vi "Stage Finished Playback.vi"(8 "error in (no error)":errorcluster, 11 "Internal Vars":T1={"Test_File"="", "Status"="Done", "RF_Center_Freq"="0", "RF_Gain"="0", "BB_Gain"="0", "Error"="", "file_max"="0", "file_index"="0"}) -> (0 "error out":errorcluster)   [LabVIEW 2017]
uses:
  TypeDef/RF Internal Data Structure (string).ctl
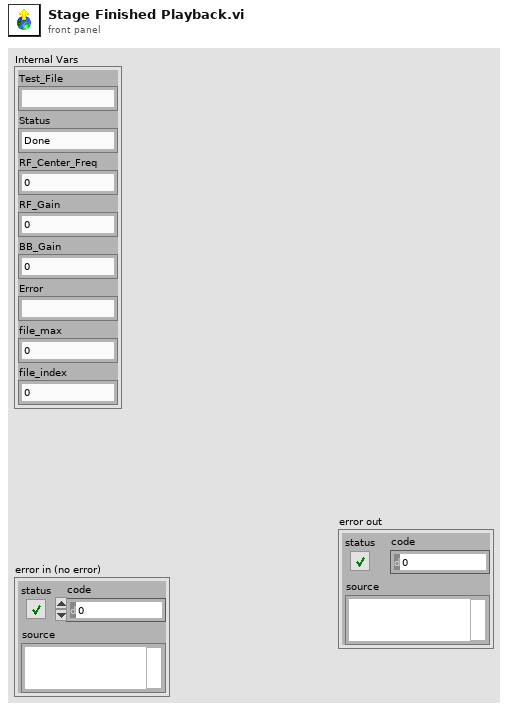
[diagram p1: front panel]
types:
  T1 = typedef "RF Internal Data Structure (string).ctl" = cluster{"Test_File":string, "Status":string, "RF_Center_Freq":string, "RF_Gain":string, "BB_Gain":string, "Error":string, "file_max":string, "file_index":string}
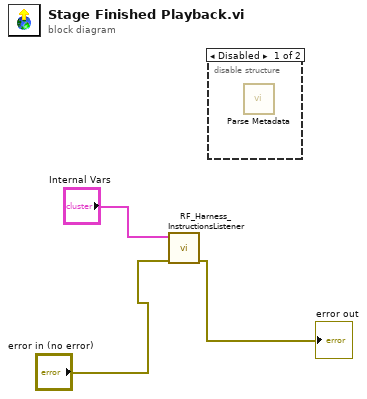
[diagram p0: block diagram]
diagram:
  n1 = call "RF_Harness_InstructionsListener.vi"("error in (no error)"="error in (no error)", "ESC Internal Data Structure"="Internal Vars") -> ("error out"=→"error out":errorcluster)  [unwired: 7 in]
  n2 = disable-structure shown="Disabled" {
    frame Disabled {
      n3 = call "Parse Metadata.vi"() -> ()  [unwired: 10 in, 2 out]
    }
    frame Enabled {
    }
  }
